vi "RO from WL and mode.vi"(9 "Mode":u8, 11 "Wavelength":u8) -> (3 "SLM pattern":u8)   [LabVIEW 2018]
panel:
  in  "Pattern array":u8[][](array[numeric])=[[4, 4, 5], [3, 4, 4], [1, 1, 2], [0, 1, 1]] step=1
  # "488           561            640"
  # "W/f\n\nTIRF\n\nSIM\n\nT-SIM"
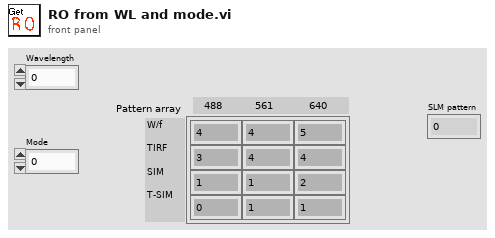
[diagram p1: front panel]
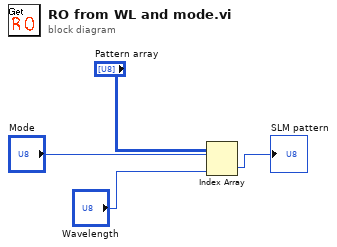
[diagram p0: block diagram]
diagram:
  n1 = Index Array(array="Pattern array", index (row)="Mode", index (col)="Wavelength") -> (element=→"SLM pattern":u8)
